vi "New Client.vi"() -> ()   [LabVIEW 2014]
uses:
  <vilib>/LabVIEW Open Source Project/MQTT Connection/MQTT_Base/Base Class/Public Events -- cluster.ctl
  <vilib>/LabVIEW Open Source Project/MQTT Control Packets/Control Packets/PUBLISH/PUBLISH.lvclass
  <vilib>/LabVIEW Open Source Project/MQTT Control Packets/Control Packets/CONNECT/ConnectFlags -- cluster.ctl
  <vilib>/LabVIEW Open Source Project/MQTT TCP Connection/MQTT_TCP/Connection/TCPConnection.lvclass
  <vilib>/LabVIEW Open Source Project/MQTT Client/Client class/Client.lvclass
  <vilib>/LabVIEW Open Source Project/MQTT Connection/MQTT_Base/Base Class/MQTT_Base.lvclass
  <vilib>/LabVIEW Open Source Project/MQTT Control Packets/Control Packets/ControlPacket/ControlPacket.lvclass
  <vilib>/LabVIEW Open Source Project/MQTT Connection/MQTT_Connection/Connection/Connection.lvclass
  <vilib>/LabVIEW Open Source Project/MQTT Control Packets/Control Packets/CONNECT/CONNECT.lvclass
panel:
  out "error out 3":errorcluster
  in  "Topic Name (empty: Payload name)":string="v1/devices/me/telemetry/Test"
  in  "text":string="{\"Test\":\"555\"}"
  out "Published 2":bool
  out "Incoming Message":u8[](array[numeric]) format="%08b"
  in  "Subscribe":bool
  out "Suback":bool
  out "Published":bool
  in  "Publish":bool
  in  "Stop Client":bool
  out "error out 2":errorcluster
  out "MQTT Public Events":T1
  out "error out":errorcluster
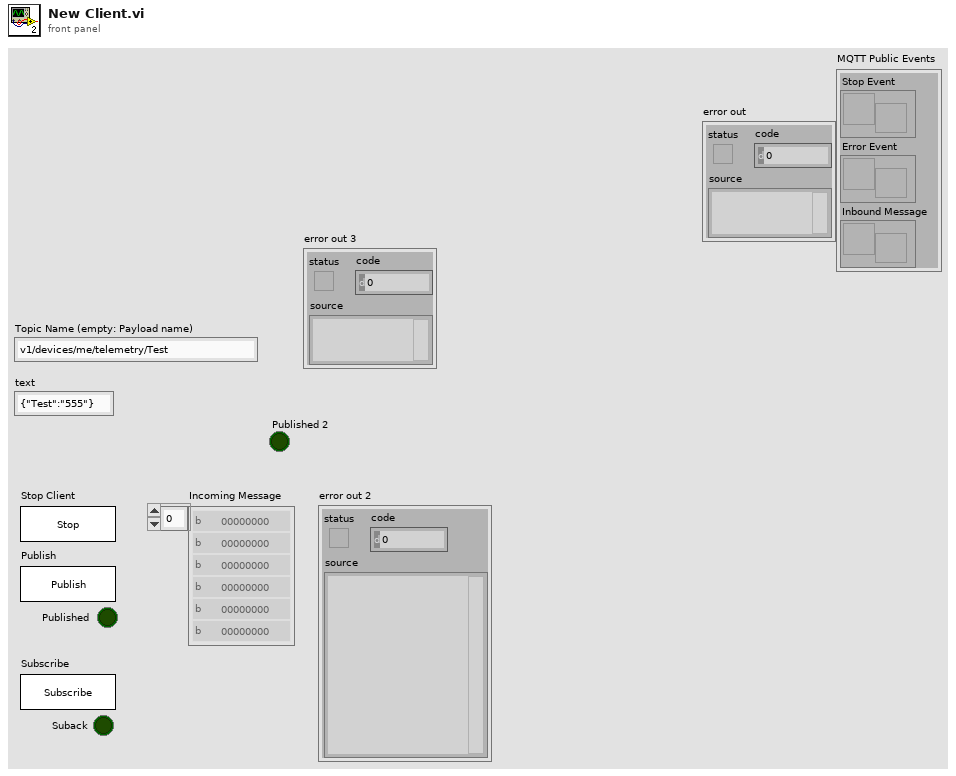
[diagram p1: front panel]
types:
  T1 = typedef "MQTT Base.lvlib/MQTT_Base.lvclass/Public Events -- cluster.ctl" = cluster{"Stop Event":refnum<user-event>, "Error Event":refnum<user-event>, "Inbound Message":refnum<user-event>}
  T2 = typedef "MQTT_Control_Packets.lvlib/CONNECT.lvclass/ConnectFlags -- cluster.ctl" = cluster{"Reserved":bool, "Clean Session":bool, "Will Flag":bool, "Will QoS 1":bool, "Will QoS 2":bool, "Will Retain":bool, "Password Flag":bool, "User Name Flag":bool}
  T3 = cluster{"Will Topic":string, "Will Message":string, "Username":string, "Password":string}[]
  T4 = typedef "MQTT Client.lvlib/Client.lvclass/Public Events -- cluster.ctl" = cluster{"Connection Status":refnum<user-event>, "Connected":refnum<user-event>, "Application Message":refnum<user-event>}
  T5 = cluster{"Will Topic":string, "Will Message":string, "Username":string, "Password":string}
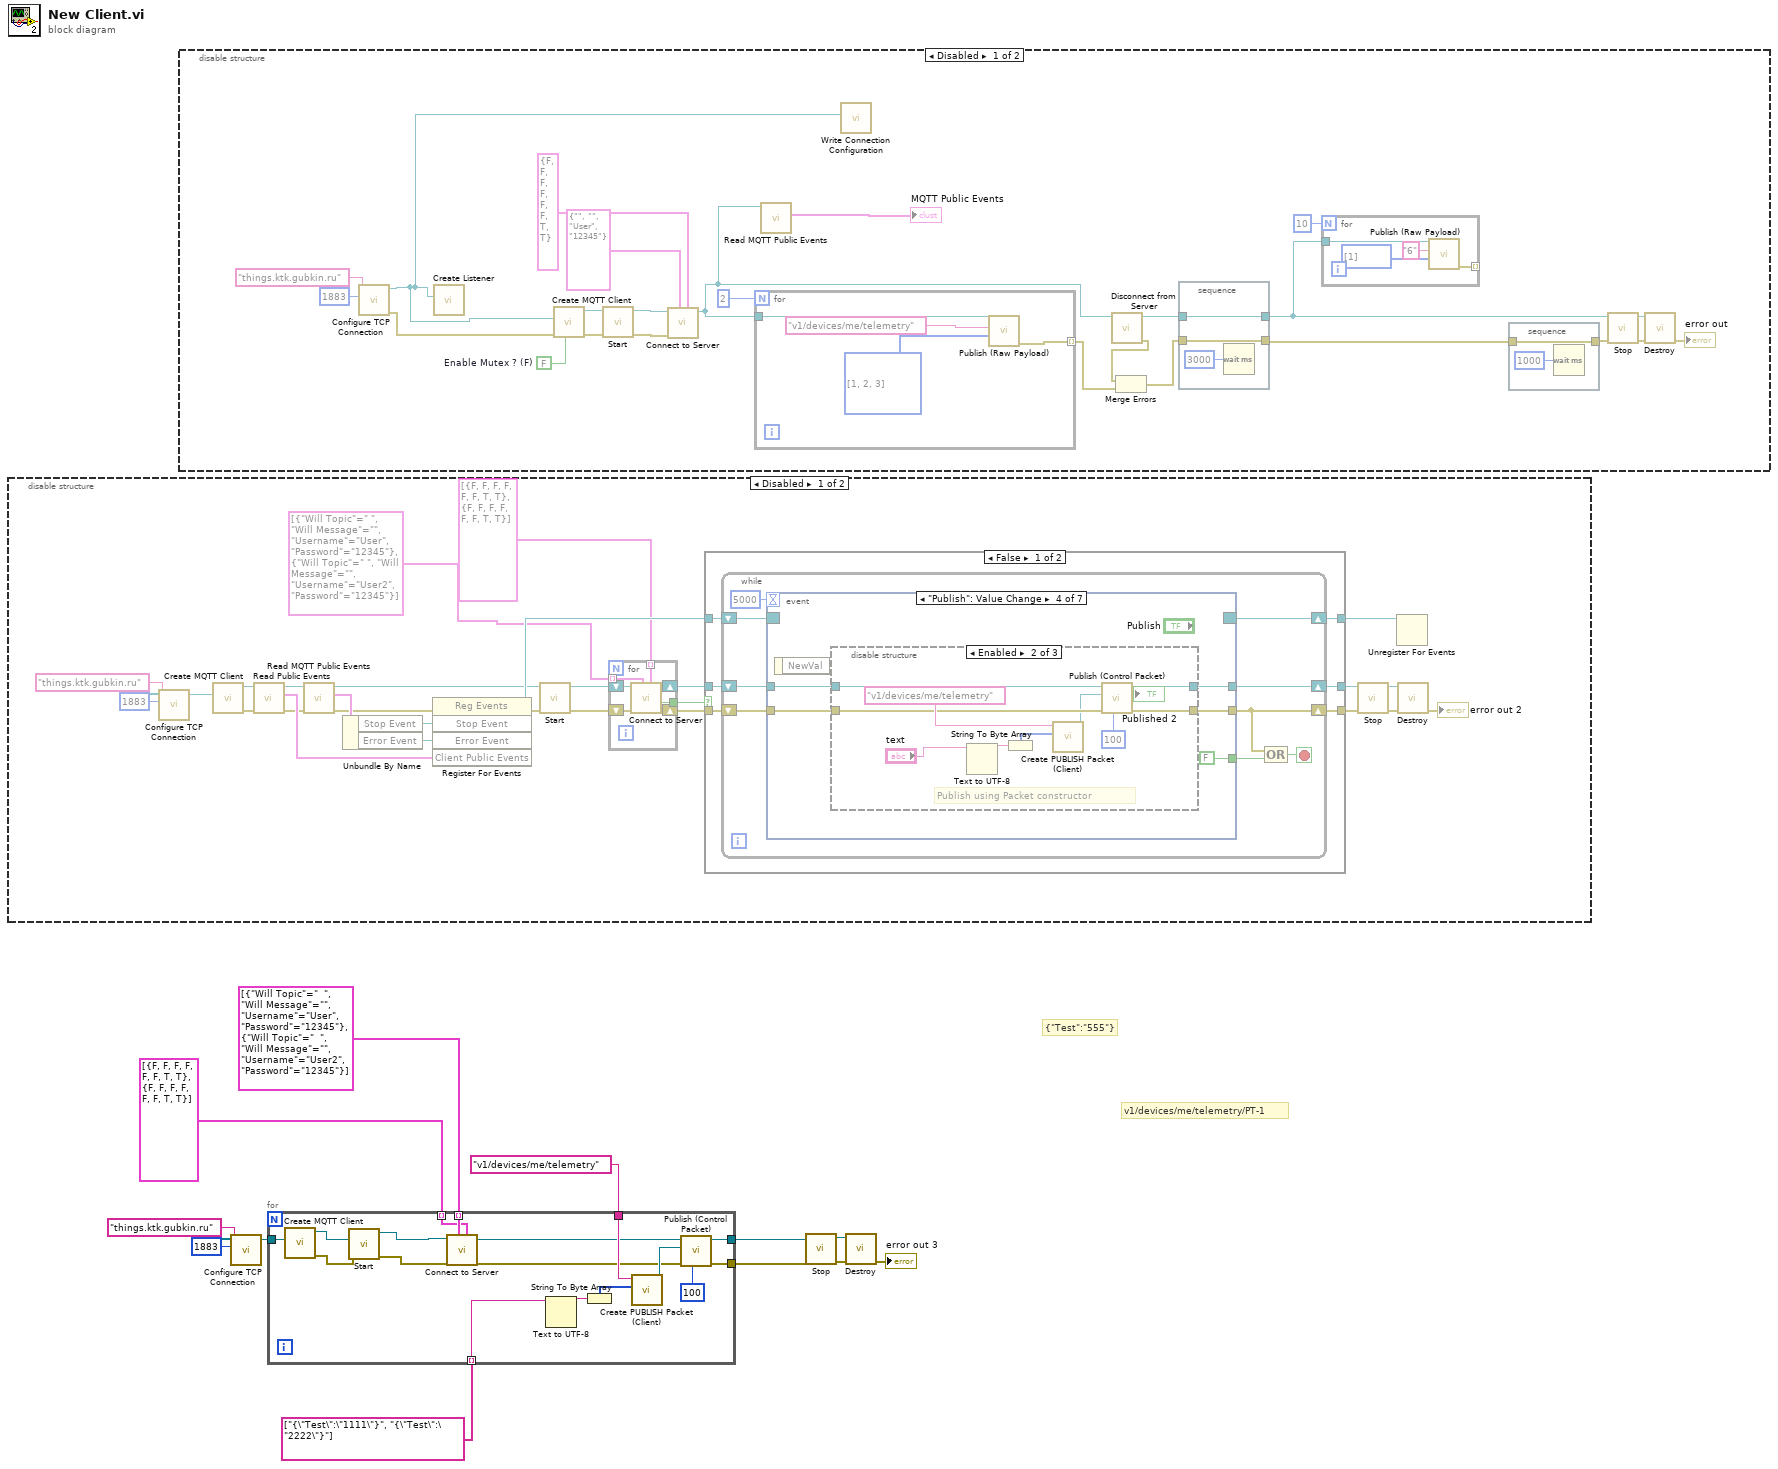
[diagram p0: block diagram]
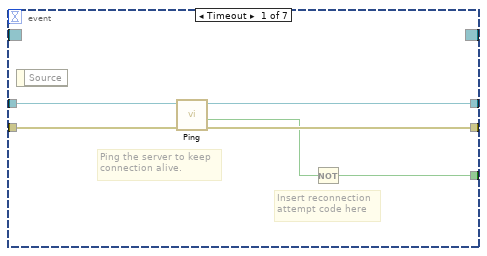
[diagram p2: hidden frame]
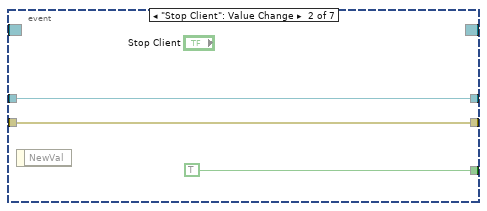
[diagram p3: hidden frame]
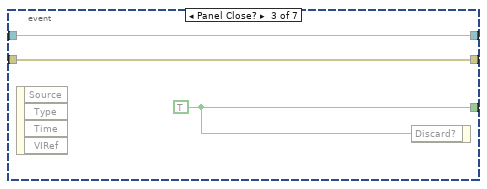
[diagram p4: hidden frame]
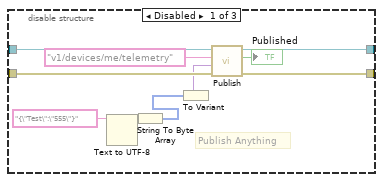
[diagram p5: hidden frame]
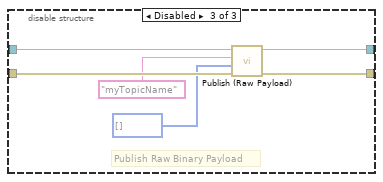
[diagram p6: hidden frame]
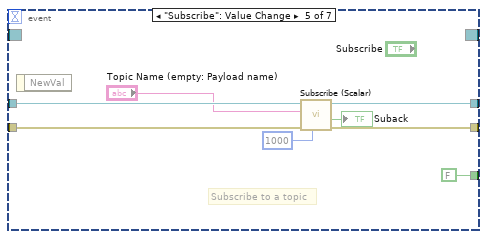
[diagram p7: hidden frame]
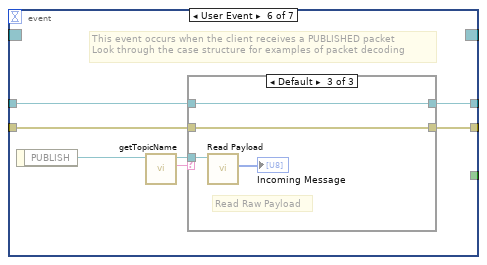
[diagram p8: hidden frame]
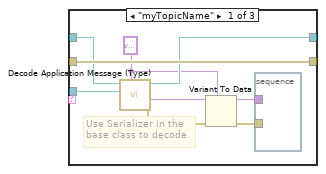
[diagram p9: hidden frame]
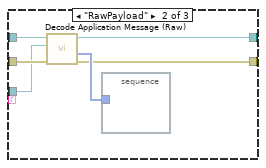
[diagram p10: hidden frame]
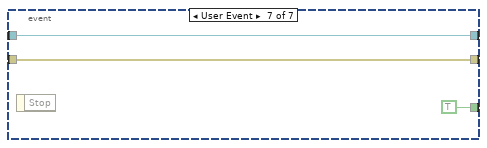
[diagram p11: hidden frame]
diagram:
  # "v1/devices/me/telemetry/PT-1"
  # "{\"Test\":\"555\"}"
  n1 = disable-structure shown="Disabled" {
    frame Disabled {
      n2 = call <vilib>:"Configure TCP Connection.vi"("remote port (80)"=u16 1883, "address (localhost)"="things.ktk.gubkin.ru") -> ("TCPConnection"=w15:refnum<class "TCPConnection.lvclass">)  [unwired: 8 in, 1 out]
      n3 = call <vilib>:"Create MQTT Client.vi"("Connection Configuration"=w15) -> ("error out"=w20:errorcluster, "Client out"=w18:refnum<class "Client.lvclass">)  [unwired: 9 in]
      n4 = call <vilib>:"Read Public Events.vi"("error in (no error)"=w20, "Client in"=w18) -> ("error out"=w21:errorcluster, "Client Public Events"=w23:T4, "Client out"=w19:refnum<class "Client.lvclass">)  [unwired: 7 in]
      n5 = call <vilib>:"Read MQTT Public Events.vi"("error in (no error)"=w21, "MQTT_Base in"=w19) -> ("error out"=w22:errorcluster, "MQTT Public Events"=w35:T1, "MQTT_Base out"=w25:refnum<class "Client.lvclass">)  [unwired: 7 in]
      n6 = Unbundle By Name(w35) -> ("Stop Event"=w33:refnum<user-event>, "Error Event"=w34:refnum<user-event>)
      n7 = register-events(error in=w22, w33, w34, w23) -> (reference out=w28:refnum<event-registration>, error out=w24:errorcluster)  [unwired: 1 in]
      n8 = call <vilib>:"Start.vi"("error in (no error)"=w24, "MQTT_Base in"=w25) -> ("error out"=w27:errorcluster, "MQTT_Base out"=w26:refnum<class "Client.lvclass">)  [unwired: 7 in, 1 out]
      n9 = for {
        tunnel: [w45] -> w30
        tunnel: T2[] [{"Reserved"=FALSE, "Clean Session"=FALSE, "Will Flag"=FALSE, "Will QoS 1"=FALSE, "Will QoS 2"=FALSE, "Will Retain"=FALSE, "Password Flag"=TRUE, "User Name Flag"=TRUE}, {"Reserved"=FALSE, "Clean Session"=FALSE, "Will Flag"=FALSE, "Will QoS 1"=FALSE, "Will QoS 2"=FALSE, "Will Retain"=FALSE, "Password Flag"=TRUE, "User Name Flag"=TRUE}] -> [w42] mode=indexing
        tunnel: T3 [{"Will Topic"=" ", "Will Message"="", "Username"="User", "Password"="12345"}, {"Will Topic"=" ", "Will Message"="", "Username"="User2", "Password"="12345"}] -> [w41] mode=indexing
        shift-right: [w46] -> w31
        shift-left: w27 -> [w44]
        shift-right: [w47] -> w32
        shift-left: w26 -> [w43]
        n10 = call <vilib>:"Connect to Server.vi"("Connect Flags"=w42, "Payload"=w41, "error in (no error)"=w44, "Client in"=w43) -> ("error out"=w46:errorcluster, "timed out"=w45:bool, "Client out"=w47:refnum<class "Client.lvclass">)  [unwired: 4 in, 1 out]
      }
      n11 = case shown="False" w30 {
        tunnel: w28 -> [w53 w146]
        tunnel: [w52 w146] -> w29
        tunnel: w31 -> [w49 w144]
        tunnel: w32 -> [w51 w145]
        tunnel: [w50 w145] -> w37
        tunnel: [w48 w144] -> w39
        frame False {
          n12 = while {
            shift-right: [w61] -> w52
            shift-left: w53 -> [w62]
            shift-right: [w54] -> w50
            shift-left: w51 -> [w55]
            shift-right: [w59] -> w48
            shift-left: w49 -> [w60]
            stop <- w58 stop-if-true
            n13 = event shown="[3] \"Publish\": Value Change" {
              selector: w62 -> [_ _ _ _ _ _ _]
              dyn-events: [_ _ _ _ _ _ _] -> w61
              timeout: 5000 -> [_ _ _ _ _ _ _]
              tunnel: w60 -> [w67 w70 w72 w77 w111 w116 w143]
              tunnel: [w65 w70 w72 w76 w110 w117 w143] -> w59
              tunnel: [w64 TRUE w74 FALSE FALSE _ TRUE] -> w57
              tunnel: w55 -> [w68 w71 w73 w78 w113 w119 w141]
              tunnel: [w66 w71 w73 w75 w109 w118 w141] -> w54
              event Timeout {
                # "Insert reconnection\nattempt code here"
                # "Ping the server to keep\nconnection alive."
                n14 = event-data() -> ()  [unwired: 1 in, 1 out]
                n15 = call <vilib>:"Ping.vi"("error in (no error)"=w67, "Client in"=w68) -> ("error out"=w65:errorcluster, "Server responded"=w63:bool, "Client out"=w66:refnum<class "Client.lvclass">)  [unwired: 6 in, 1 out]
                n16 = Not(x=w63) -> (.not. x?=w64:bool)
              }
              event "Stop Client": Value Change {
                n17 = event-data() -> ()  [unwired: 1 in, 1 out]
              }
              event Panel Close? {
                w74 = TRUE
                n18 = event-data() -> ()  [unwired: 1 in, 4 out]
                n19 = event-data("Discard?"=w74) -> ()  [unwired: 1 in, 1 out]
              }
              event "Publish": Value Change {
                n20 = event-data() -> ()  [unwired: 1 in, 1 out]
                n21 = disable-structure shown="Enabled" {
                  disable-tunnel: w78 -> [w89 w99 w106]
                  disable-tunnel: w77 -> [w88 w98 w103]
                  disable-tunnel: [w87 w97 w104] -> w76
                  disable-tunnel: [w86 w90 w105] -> w75
                  frame Disabled {
                    # "Publish Anything"
                    n22 = Text to UTF-8(11:"{\"Test\":\"555\"}" ("text")) -> (3:w82:string)  [unwired: 2 in, 1 out]
                    n23 = String To Byte Array(string=w82) -> (unsigned byte array=w81:u8[])
                    n24 = To Variant(anything=w81) -> (Variant=w84:variant)
                    n25 = call <vilib>:"Publish.vi"("error in (no error)"=w88, "Payload"=w84, "Topic Name (empty: Payload name)"="v1/devices/me/telemetry", "Client in"=w89) -> ("error out"=w87:errorcluster, "Published"=→"Published":bool, "Client out"=w86:refnum<class "Client.lvclass">)  [unwired: 5 in]
                  }
                  frame Enabled {
                    # "Publish using Packet constructor"
                    n26 = Text to UTF-8(11:"text") -> (3:w93:string)  [unwired: 2 in, 1 out]
                    n27 = String To Byte Array(string=w93) -> (unsigned byte array=w91:u8[])
                    n28 = call <vilib>:"Create PUBLISH Packet (Client).vi"("Payload"=w91, "Topic Name"="v1/devices/me/telemetry" ("Topic Name (empty: Payload name)")) -> ("PUBLISH"=w95:refnum<class "PUBLISH.lvclass">)  [unwired: 6 in, 3 out]
                    n29 = call <vilib>:"Publish (Control Packet).vi"("timeout (1000ms)"=100 ("timeout (0ms : no ack)"), "error in (no error)"=w98, "PUBLISH"=w95, "Client in"=w99) -> ("error out"=w97:errorcluster, "Published"=→"Published 2":bool, "Client out"=w90:refnum<class "Client.lvclass">)  [unwired: 5 in]
                  }
                  frame Disabled {
                    # "Publish Raw Binary Payload"
                    n30 = call <vilib>:"Publish (Raw Payload).vi"("error in (no error)"=w103, "Binary Payload"=u8[] [] ("Payload"), "Topic Name"="myTopicName" ("Topic Name (empty: Payload name)"), "Client in"=w106) -> ("error out"=w104:errorcluster, "Client out"=w105:refnum<class "Client.lvclass">)  [unwired: 5 in, 1 out]
                  }
                }
              }
              event "Subscribe": Value Change {
                # "Subscribe to a topic"
                n31 = event-data() -> ()  [unwired: 1 in, 1 out]
                n32 = call <vilib>:"Subscribe (Scalar).vi"("timeout (1000ms)"=1000 ("timeout (100ms)"), "error in (no error)"=w111, "Topic Filter"="Topic Name (empty: Payload name)", "Client in"=w113) -> ("error out"=w110:errorcluster, "Ack"=→"Suback":bool, "Client out"=w109:refnum<class "Client.lvclass">)  [unwired: 5 in]
              }
              event User Event {
                # "This event occurs when the client receives a PUBLISHED packet\nLook through the case structure for examples of packet decoding"
                n33 = event-data() -> ("PUBLISH"=w121:refnum<class "PUBLISH.lvclass">)  [unwired: 1 in]
                n34 = call <vilib>:"getTopicName.vi"("PUBLISH in"=w121) -> ("Topic"=w120:string, "PUBLISH out"=w115:refnum<class "PUBLISH.lvclass">)  [unwired: 8 in, 1 out]
                n35 = case shown="Default" w120 {
                  tunnel: w119 -> [w127 w136 w140]
                  tunnel: [w126 w135 w140] -> w118
                  tunnel: [w130 w133 w139] -> w117
                  tunnel: w116 -> [w130 w132 w139]
                  tunnel: w115 -> [w125 w131 w138]
                  frame "myTopicName" {
                    w123 = variant ("Type")
                    # "Use Serializer in the\nbase class to decode"
                    n36 = call <vilib>:"Decode Application Message (Type).vi"("Type"=w123, "PUBLISH"=w125, "Client in"=w127) -> ("error out"=w122:errorcluster, "Payload"=w124:variant, "Client out"=w126:refnum<class "Client.lvclass">)  [unwired: 5 in, 1 out]
                    n37 = Variant To Data(error in=w122, type=w123, Variant=w124) -> (data=w129:variant, error out=w128:errorcluster)
                    n38 = stacked-sequence {
                      tunnel: w129 -> [_]
                      tunnel: w128 -> [_]
                      frame #0 {
                      }
                    }
                  }
                  frame "RawPayload" {
                    n39 = call <vilib>:"Decode Application Message (Raw).vi"("error in (no error)"=w132, "PUBLISH"=w131, "Client in"=w136) -> ("error out"=w133:errorcluster, "Payload"=w134:u8[], "Client out"=w135:refnum<class "Client.lvclass">)  [unwired: 5 in, 1 out]
                    n40 = stacked-sequence {
                      tunnel: w134 -> [_]
                      frame #0 {
                      }
                    }
                  }
                  frame Default {
                    # "Read Raw Payload"
                    n41 = call <vilib>:"Read Payload.vi"("ControlPacket in"=w138) -> ("Payload"=→"Incoming Message":u8[])  [unwired: 9 in, 1 out]
                  }
                }
              }
              event User Event {
                n42 = event-data() -> ()  [unwired: 1 in, 1 out]
              }
            }
            n43 = Compound Arithmetic op=OR(w59, w57) -> (w58:bool)
          }
        }
        frame True {
        }
      }
      n44 = call <vilib>:"Stop.vi"("error in (no error)"=w39, "MQTT_Base in"=w37) -> ("error out"=w38:errorcluster, "MQTT_Base out"=w36:refnum<class "Client.lvclass">)  [unwired: 7 in, 1 out]
      n45 = Unregister For Events(event registration refnum=w29) -> ()  [unwired: 1 in, 1 out]
      n46 = call <vilib>:"Destroy.vi"("error in (no error)"=w38, "MQTT_Base in"=w36) -> ("error out"=→"error out 2":errorcluster)  [unwired: 8 in, 1 out]
    }
    frame Enabled {
    }
  }
  n47 = disable-structure shown="Disabled" {
    frame Disabled {
      w170 = FALSE  # Enable Mutex ? (F)
      n48 = call <vilib>:"Configure TCP Connection.vi"("remote port (80)"=u16 1883, "address (localhost)"="things.ktk.gubkin.ru") -> ("error out"=w156:errorcluster, "TCPConnection"=w148:refnum<class "TCPConnection.lvclass">)  [unwired: 8 in]
      n49 = call <vilib>:"Create Listener.vi"("Connection Configuration"=w148) -> ()  [unwired: 9 in, 2 out]
      n50 = call <vilib>:"Create MQTT Client.vi"("Enable Mutex ? (F)"=w170, "error in (no error)"=w156, "Connection Configuration"=w148) -> ("error out"=w166:errorcluster, "Client out"=w168:refnum<class "Client.lvclass">)  [unwired: 7 in]
      n51 = call <vilib>:"Start.vi"("error in (no error)"=w166, "MQTT_Base in"=w168) -> ("error out"=w167:errorcluster, "MQTT_Base out"=w169:refnum<class "Client.lvclass">)  [unwired: 7 in, 1 out]
      n52 = call <vilib>:"Connect to Server.vi"("Connect Flags"=T2 {"Reserved"=FALSE, "Clean Session"=FALSE, "Will Flag"=FALSE, "Will QoS 1"=FALSE, "Will QoS 2"=FALSE, "Will Retain"=FALSE, "Password Flag"=TRUE, "User Name Flag"=TRUE}, "Payload"=T5 {"Will Topic"="", "Will Message"="", "Username"="User", "Password"="12345"}, "error in (no error)"=w167, "Client in"=w169) -> ("Client out"=w150:refnum<class "Client.lvclass">)  [unwired: 4 in, 3 out]
      n53 = for {
        N: 2 -> [_]
        tunnel: w150 -> [w183]
        tunnel: [w182] -> w153 mode=indexing
        n54 = call <vilib>:"Publish (Raw Payload).vi"("Binary Payload"=u8[] [1, 2, 3], "Topic Name"="v1/devices/me/telemetry", "Client in"=w183) -> ("error out"=w182:errorcluster)  [unwired: 6 in, 2 out]
      }
      n55 = call <vilib>:"Read MQTT Public Events.vi"("MQTT_Base in"=w150) -> ("MQTT Public Events"=→"MQTT Public Events":T1)  [unwired: 8 in, 2 out]
      n56 = call <vilib>:"Write Connection Configuration.vi"("Connection Configuration"=w148) -> ("MQTT_Base in"=w147:refnum<class "MQTT_Base.lvclass">)  [unwired: 8 in, 2 out]
      n57 = call <vilib>:"Disconnect from Server.vi"("Client in"=w150) -> ("error out"=w152:errorcluster, "Client out"=w157:refnum<class "Client.lvclass">)  [unwired: 8 in, 1 out]
      n58 = Merge Errors(w152, w153) -> (w151:errorcluster)
      n59 = stacked-sequence {
        tunnel: w151 -> [w180]
        tunnel: [w180] -> w159
        tunnel: [w179] -> w158
        tunnel: w157 -> [w179]
        frame #0 {
          n60 = Wait (ms)(milliseconds to wait=u32 3000) -> ()  [unwired: 1 out]
        }
      }
      n61 = for {
        N: 10 -> [_]
        tunnel: w158 -> [w176]
        tunnel: [w175] -> _ mode=indexing
        n62 = call <vilib>:"Publish (Raw Payload).vi"("Binary Payload"=u8[] [1], "Topic Name"="6", "Client in"=w176) -> ("error out"=w175:errorcluster)  [unwired: 6 in, 2 out]
      }
      n63 = stacked-sequence {
        tunnel: w159 -> [w173]
        tunnel: [w173] -> w160
        frame #0 {
          n64 = Wait (ms)(milliseconds to wait=u32 1000) -> ()  [unwired: 1 out]
        }
      }
      n65 = call <vilib>:"Stop.vi"("error in (no error)"=w160, "MQTT_Base in"=w158) -> ("error out"=w162:errorcluster, "MQTT_Base out"=w163:refnum<class "Client.lvclass">)  [unwired: 7 in, 1 out]
      n66 = call <vilib>:"Destroy.vi"("error in (no error)"=w162, "MQTT_Base in"=w163) -> ("error out"=→"error out":errorcluster)  [unwired: 8 in, 1 out]
    }
    frame Enabled {
    }
  }
  n67 = call <vilib>:"Configure TCP Connection.vi"("remote port (80)"=u16 1883, "address (localhost)"="things.ktk.gubkin.ru") -> ("TCPConnection"=w2:refnum<class "TCPConnection.lvclass">)  [unwired: 8 in, 1 out]
  n68 = for {
    tunnel: "v1/devices/me/telemetry" ("Topic Name (empty: Payload name)") -> [w202]
    tunnel: [w201] -> w8
    tunnel: [w200] -> w7
    tunnel: T3 [{"Will Topic"="  ", "Will Message"="", "Username"="User", "Password"="12345"}, {"Will Topic"="  ", "Will Message"="", "Username"="User2", "Password"="12345"}] -> [w199] mode=indexing
    tunnel: T2[] [{"Reserved"=FALSE, "Clean Session"=FALSE, "Will Flag"=FALSE, "Will QoS 1"=FALSE, "Will QoS 2"=FALSE, "Will Retain"=FALSE, "Password Flag"=TRUE, "User Name Flag"=TRUE}, {"Reserved"=FALSE, "Clean Session"=FALSE, "Will Flag"=FALSE, "Will QoS 1"=FALSE, "Will QoS 2"=FALSE, "Will Retain"=FALSE, "Password Flag"=TRUE, "User Name Flag"=TRUE}] -> [w198] mode=indexing
    tunnel: w2 -> [w197]
    tunnel: string[] ["{\"Test\":\"1111\"}", "{\"Test\":\"2222\"}"] -> [w186] mode=indexing
    n69 = call <vilib>:"Create MQTT Client.vi"("Connection Configuration"=w197) -> ("error out"=w195:errorcluster, "Client out"=w196:refnum<class "Client.lvclass">)  [unwired: 9 in]
    n70 = call <vilib>:"Start.vi"("error in (no error)"=w195, "MQTT_Base in"=w196) -> ("error out"=w193:errorcluster, "MQTT_Base out"=w194:refnum<class "Client.lvclass">)  [unwired: 7 in, 1 out]
    n71 = call <vilib>:"Connect to Server.vi"("Connect Flags"=w198, "Payload"=w199, "error in (no error)"=w193, "Client in"=w194) -> ("error out"=w187:errorcluster, "Client out"=w188:refnum<class "Client.lvclass">)  [unwired: 4 in, 2 out]
    n72 = Text to UTF-8(11:w186) -> (3:w191:string)  [unwired: 2 in, 1 out]
    n73 = String To Byte Array(string=w191) -> (unsigned byte array=w192:u8[])
    n74 = call <vilib>:"Create PUBLISH Packet (Client).vi"("Payload"=w192, "Topic Name"=w202) -> ("PUBLISH"=w190:refnum<class "PUBLISH.lvclass">)  [unwired: 6 in, 3 out]
    n75 = call <vilib>:"Publish (Control Packet).vi"("timeout (1000ms)"=100 ("timeout (0ms : no ack)"), "error in (no error)"=w187, "PUBLISH"=w190, "Client in"=w188) -> ("error out"=w200:errorcluster, "Client out"=w201:refnum<class "Client.lvclass">)  [unwired: 5 in, 1 out]
  }
  n76 = call <vilib>:"Stop.vi"("error in (no error)"=w7, "MQTT_Base in"=w8) -> ("error out"=w9:errorcluster, "MQTT_Base out"=w6:refnum<class "Client.lvclass">)  [unwired: 7 in, 1 out]
  n77 = call <vilib>:"Destroy.vi"("error in (no error)"=w9, "MQTT_Base in"=w6) -> ("error out"=→"error out 3":errorcluster)  [unwired: 8 in, 1 out]
